vi "Inverse Kinematics Trajectory Visualizer.vi"(9 "dt":dbl, 10 "Target Velocity":cluster{"Vx":dbl, "Vy":dbl, "Omega":dbl}, 11 "# Points":i32) -> (3 "Points":cluster{dbl[], dbl[]})   [LabVIEW 2023]
uses:
  <vilib>/Analysis/coordinate.llb/2D Cartesian Coordinate Rotation (Scalar).vi
  <vilib>/Analysis/NI_AALPro.lvlib
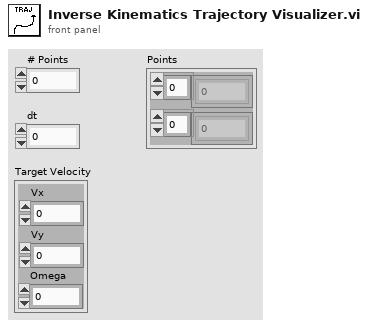
[diagram p1: front panel]
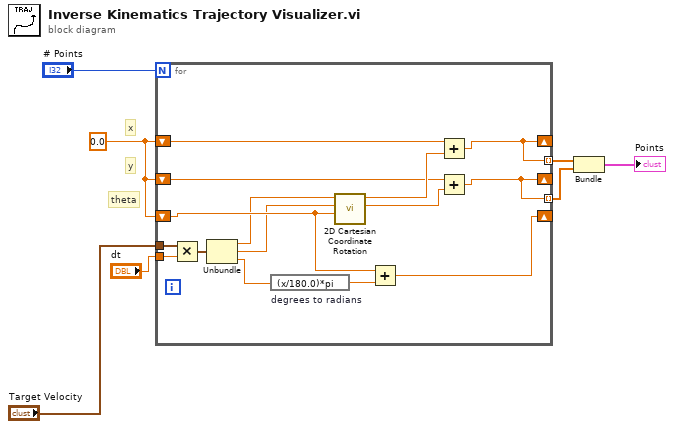
[diagram p0: block diagram]
diagram:
  w3 = 0.0 ("dt")
  # "theta"
  # "y"
  # "x"
  n1 = for {
    N: "# Points" -> [_]
    shift-right: [w13] -> _
    shift-left: w3 -> [w20]
    shift-right: [w12] -> _
    shift-left: w3 -> [w18]
    shift-right: [w14] -> _
    shift-left: w3 -> [w15]
    tunnel: "Target Velocity" -> [w22]
    tunnel: "dt" -> [w21]
    tunnel: [w13] -> w5 mode=indexing
    tunnel: [w12] -> w6 mode=indexing
    n2 = Multiply(x=w22, y=w21) -> (x*y=w11:cluster{"Vx":dbl, "Vy":dbl, "Omega":dbl})
    n3 = Unbundle(w11) -> ("Vx"=w10:dbl, "Vy"=w9:dbl, "Omega"=w8:dbl)
    n4 = expression code="(x/180.0)*pi" "degrees to radians"(w8) -> (w16:dbl)
    n5 = call-poly <vilib>:"2D Cartesian Coordinate Rotation.vi"("theta"=w15, "y"=w9, "x"=w10) -> ("y out"=w17:dbl, "x out"=w19:dbl)  [unwired: 6 in, 1 out]
    n6 = Add(x=w15, y=w16) -> (x+y=w14:dbl)
    n7 = Add(x=w20, y=w19) -> (x+y=w13:dbl)
    n8 = Add(x=w18, y=w17) -> (x+y=w12:dbl)
  }
  n9 = Bundle(w5, w6) -> (→"Points":cluster{dbl[], dbl[]})  [unwired: 1 in]
